vi "xdata_read.vi"(5 "COM":bool, 7 "VISA name":refnum<visa-resource-name>, 9 "data":u8[](array[numeric]), 10 "wLen":u16, 11 "wAddr":u16) -> (2 "data out":u8[](array[numeric]), 3 "return":i32)   [LabVIEW 2016]
panel:
  in  "vd_cmd_short_header_t":T1
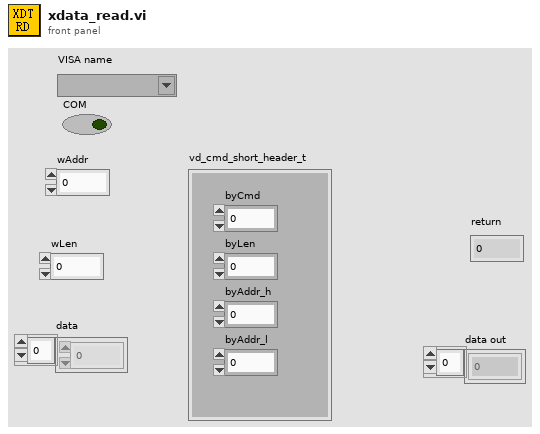
[diagram p1: front panel]
types:
  T1 = cluster{"byCmd":u8, "byLen":u8, "byAddr_h":u8, "byAddr_l":u8}
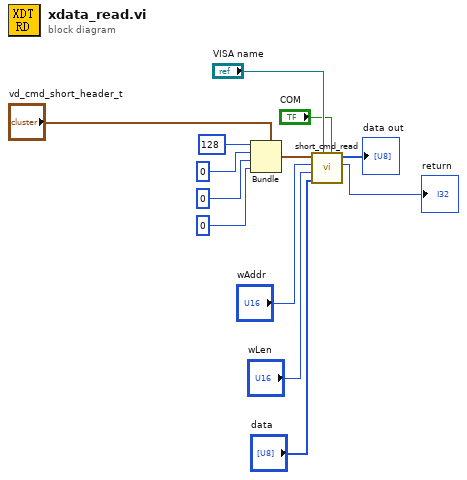
[diagram p0: block diagram]
diagram:
  n1 = Bundle(cluster="vd_cmd_short_header_t", "byCmd"=u8 128, "byLen"=u8 0, "byAddr_h"=u8 0, "byAddr_l"=u8 0) -> (w8:T1)
  n2 = call "short_cmd_read.vi"("COM"="COM", "VISA name"="VISA name", "data"="data", "dwLen"="wLen", "dwAddr"="wAddr", "cmd_short_header_t"=w8) -> ("return"=→"return":i32, "data out"=→"data out":u8[])  [unwired: 4 in]
